vi "OpenIniInNotepad.vi"(11 "Path":path) -> ()   [LabVIEW 2014]
panel:
  out "error out":errorcluster
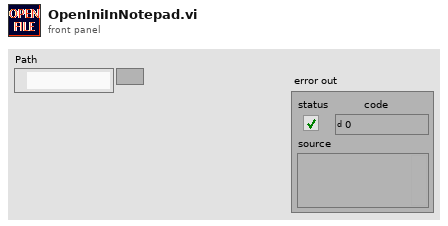
[diagram p1: front panel]
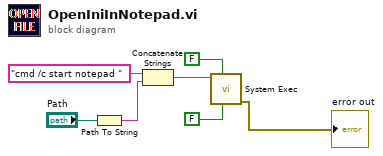
[diagram p0: block diagram]
diagram:
  n1 = Path To String(path="Path") -> (string=w4:string)
  n2 = Concatenate Strings("cmd /c start notepad " ("command line"), w4) -> (w2:string)
  n3 = call <vilib>:"System Exec.vi"("run minimized? (F)"=FALSE, "wait until completion? (T)"=FALSE, "command line"=w2) -> ("error out"=→"error out":errorcluster)  [unwired: 5 in, 3 out]
